vi "Match Regex.vi"(7 "regular expression":string, 8 "error in (no error)":errorcluster, 9 "offset":i32, 11 "String":string) -> (0 "error out":errorcluster, 1 "offset past match":i32, 2 "submatch 1":string, 3 "whole match":string)   [LabVIEW 2020, in "TOML.lvlib"]
uses:
  TOML.lvlib
  <vilib>/regexp/Match Regular Expression.xnode
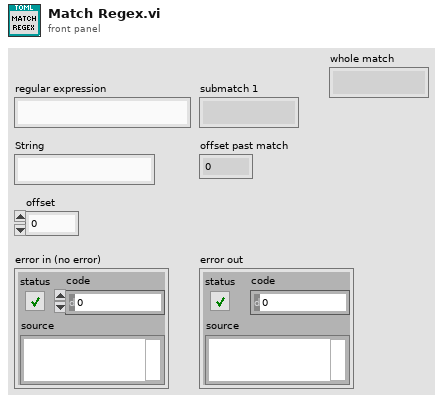
[diagram p1: front panel]
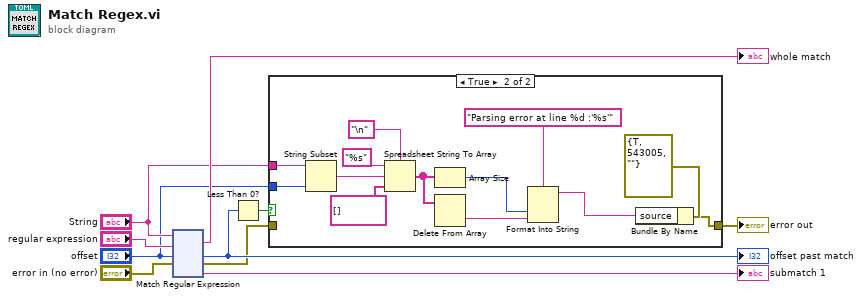
[diagram p0: block diagram]
diagram:
  n1 = xnode "Match Regular Expression"("input string"="String", "regular expression"="regular expression", "offset (0)"="offset", "error in"="error in (no error)") -> ("whole match"=→"whole match":string, "offset past match"=w9:i32, "error out"=w4:errorcluster, "submatch 1"=→"submatch 1":string)  [unwired: 2 in, 2 out]
  "offset past match" <- w9
  n2 = Less Than 0?(x=w9) -> (x < 0?=w5:bool)
  n3 = case shown="True" w5 {
    tunnel: "offset" -> [_ w18]
    tunnel: w4 -> [w11 _]
    tunnel: [w11 w13] -> w3
    tunnel: "String" -> [_ w23]
    frame False {
    }
    frame True {
      n4 = String Subset(string=w23, length (rest)=w18) -> (substring=w21:string)  [unwired: 1 in]
      n5 = Spreadsheet String To Array(delimiter (Tab)="\n", format string="%s" ("delimiter (Tab)"), spreadsheet string=w21, array type (2D Dbl)=string[] []) -> (array=w16:string[])
      n6 = Array Size(array=w16) -> (size(s)=w17:i32)
      n7 = Delete From Array(array=w16) -> (deleted portion=w15:string)  [unwired: 2 in, 1 out]
      n8 = Format Into String(format string="Parsing error at line %d :'%s'", w17, w15) -> (resulting string=w12:string)  [unwired: 2 in, 1 out]
      n9 = Bundle By Name(cluster=errorcluster {"status"=TRUE, "code"=543005, "source"=""} ("error out"), "source"=w12) -> (w13:errorcluster)
    }
  }
  "error out" <- w3
